vi "aquire single subvi.vi"(8 "Channel":enum16{"Invalid", "Channel 1", "Channel 2"}(ring), 9 "Array":string[](array[string])=["0", "50mv", "100mv", "200mv", "500mv", "1v", "2v", "5v", "10v", "20v", "50v", "0", "0", "0", "0", "0", "0", "0", "0", "0"], 10 "Array 3":string[](array[string])=["5ns", "10ns", "20ns", "50ns", "100ns", "200ns", "500ns", "1us", "2us", "5us", "10us", "20us", "50us", "100us", "200us", "500us", "1ms", "2ms", "5ms", "10ms", "20ms", "50ms", "100ms", "200ms", "500ms", "1s", "2s", "5s", "10s", "20s", "50s", "100s"], 11 "unsigned byte array":u8[](array[numeric])) -> (0 "wave_data(mv)":i32[](array[numeric]), 1 "M":string, 2 "precision":string, 3 "wave_data":i8[](array[numeric]))   [LabVIEW 2023, in "owon.lvlib"]
uses:
  owon.lvlib
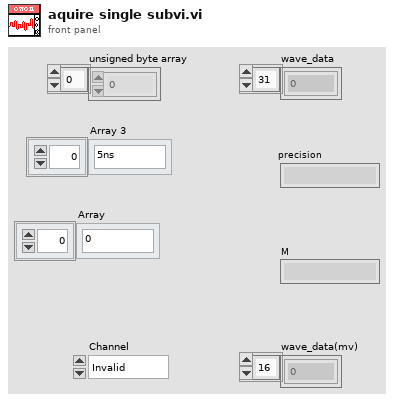
[diagram p1: front panel]
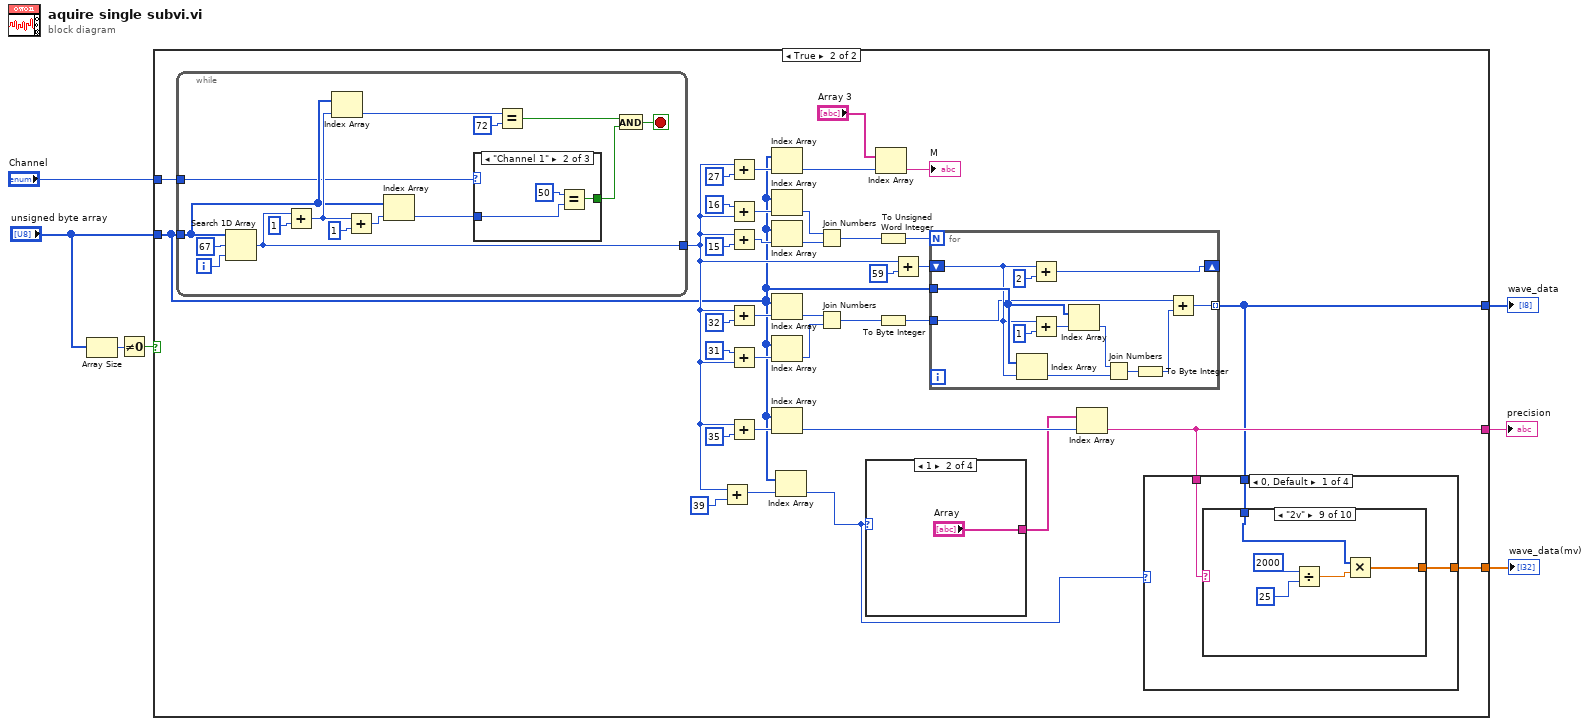
[diagram p0: block diagram]
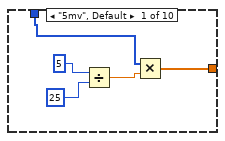
[diagram p3: hidden frame]
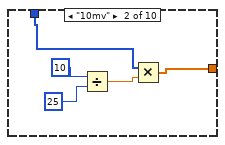
[diagram p4: hidden frame]
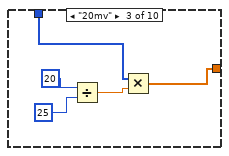
[diagram p5: hidden frame]
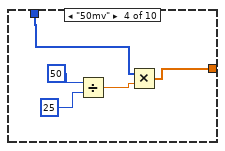
[diagram p6: hidden frame]
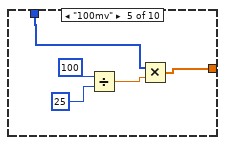
[diagram p7: hidden frame]
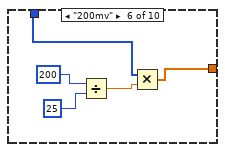
[diagram p8: hidden frame]
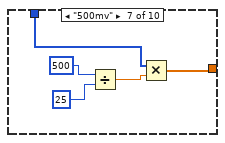
[diagram p9: hidden frame]
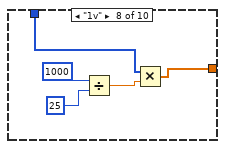
[diagram p10: hidden frame]
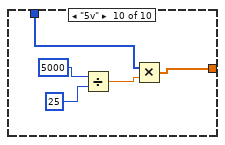
[diagram p11: hidden frame]
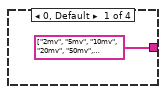
[diagram p15: hidden frame]
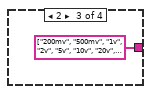
[diagram p16: hidden frame]
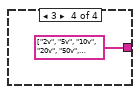
[diagram p17: hidden frame]
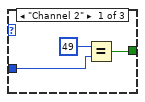
[diagram p18: hidden frame]
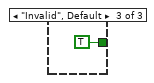
[diagram p19: hidden frame]
diagram:
  n1 = Array Size(array="unsigned byte array") -> (size(s)=w2:i32)
  n2 = Not Equal To 0?(x=w2) -> (x != 0?=w1:bool)
  n3 = case shown="True" w1 {
    tunnel: "unsigned byte array" -> [_ w14]
    tunnel: [_ w11] -> w7
    tunnel: [_ w10] -> w6
    tunnel: [_ w9] -> w5
    tunnel: "Channel" -> [_ w8]
    frame False {
    }
    frame True {
      n4 = while {
        tunnel: w14 -> [w106]
        tunnel: [w110] -> w15
        tunnel: w8 -> [w101]
        i -> [w111]
        stop <- w102 stop-if-true
        n5 = Search 1D Array(1D array=w106, element=u8 67 ("元素"), start index (0)=w111) -> (index of element=w110:i32)
        n6 = Add(x=w110, y=1) -> (x+y=w109:i32)
        n7 = Index Array(array=w106, index=w109) -> (element=w113:u8)
        n8 = Add(x=w109, y=1) -> (x+y=w107:i32)
        n9 = Index Array(array=w106, index=w107) -> (element=w105:u8)
        n10 = case shown="\"Channel 1\"" w101 {
          tunnel: w105 -> [w116 w120 _]
          tunnel: [w117 w119 TRUE] -> w104
          frame "Channel 2" {
            n11 = Equal?(x=u8 49, y=w116) -> (x = y?=w117:bool)
          }
          frame "Channel 1" {
            n12 = Equal?(x=u8 50, y=w120) -> (x = y?=w119:bool)
          }
          frame "Invalid", Default {
          }
        }
        n13 = Equal?(x=w113, y=u8 72 ("元素")) -> (x = y?=w103:bool)
        n14 = And(x=w103, y=w104) -> (x .and. y?=w102:bool)
      }
      n15 = Add(x=w15, y=39) -> (x+y=w17:i32)
      n16 = Add(x=w15, y=27) -> (x+y=w19:i32)
      n17 = Add(x=16 ("索引"), y=w15) -> (x+y=w37:i32)
      n18 = Add(x=w15, y=15 ("索引")) -> (x+y=w39:i32)
      n19 = Add(x=w15, y=32) -> (x+y=w28:i32)
      n20 = Add(x=31, y=w15) -> (x+y=w30:i32)
      n21 = Add(x=w15, y=35) -> (x+y=w22:i32)
      n22 = Index Array(array=w14, index=w19) -> (element=w18:u8)
      n23 = Index Array(array=w14, index=w37) -> (element=w40:u8)
      n24 = Index Array(array=w14, index=w39) -> (element=w41:u8)
      n25 = Index Array(array=w14, index=w28) -> (element=w25:u8)
      n26 = Index Array(array=w14, index=w30) -> (element=w26:u8)
      n27 = Index Array(array=w14, index=w22) -> (element=w21:u8)
      n28 = Index Array(array=w14, index=w17) -> (element=w12:u8)
      n29 = Join Numbers(hi=w40, lo=w41) -> ((hi.lo)=w42:u16)
      n30 = Join Numbers(hi=w25, lo=w26) -> ((hi.lo)=w24:u16)
      n31 = case shown="1" w12 {
        tunnel: [string[] ["2mv", "5mv", "10mv", "20mv", "50mv", "100mv", "200mv", "500mv", "1v", "2v", "5v", "10v", "0", "0", "0", "0", "0", "0", "0", "0"] ("Array 2") "Array" string[] ["200mv", "500mv", "1v", "2v", "5v", "10v", "20v", "50v", "100v", "200v", "500v", "1kv", "0", "0", "0", "0", "0", "0", "0", "0"] ("Array 4") string[] ["2v", "5v", "10v", "20v", "50v", "100v", "200v", "500v", "1kv", "2kv", "5kv", "10kv", "0", "0", "0", "0", "0", "0", "0", "0"] ("Array 5")] -> w13
        frame 0, Default {
        }
        frame 1 {
        }
        frame 2 {
        }
        frame 3 {
        }
      }
      n32 = Index Array(array="Array 3", index=w18) -> (element=→"M":string)
      n33 = To Unsigned Word Integer(number=w42) -> (unsigned 16bit integer=w43:u16)
      n34 = To Byte Integer(number=w24) -> (8bit integer=w33:i8)
      n35 = Add(x=w15, y=59) -> (x+y=w32:i32)
      n36 = for {
        N: w43 -> [_]
        tunnel: w14 -> [w134]
        shift-right: [w131] -> _
        shift-left: w32 -> [w130]
        tunnel: [w126] -> w10 mode=indexing
        tunnel: w33 -> [w123]
        n37 = Index Array(array=w134, index=w130) -> (element=w124:u8)
        n38 = Add(x=w130, y=2) -> (x+y=w131:i32)
        n39 = Add(x=w130, y=1) -> (x+y=w133:i32)
        n40 = Index Array(array=w134, index=w133) -> (element=w125:u8)
        n41 = Join Numbers(hi=w125, lo=w124) -> ((hi.lo)=w128:u16)
        n42 = To Byte Integer(number=w128) -> (8bit integer=w127:i8)
        n43 = Add(x=w123, y=w127) -> (x+y=w126:i8)
      }
      n44 = Index Array(array=w13, index=w21) -> (element=w11:string)
      n45 = case shown="0, Default" w12 {
        tunnel: w11 -> [w46 _ _ _]
        tunnel: w10 -> [w45 _ _ _]
        tunnel: [w44 _ _ _] -> w9
        frame 0, Default {
          n46 = case shown="\"2v\"" w46 {
            tunnel: w45 -> [w48 w53 w58 w63 w68 w73 w78 w83 w88 w93]
            tunnel: [w47 w52 w57 w62 w67 w72 w77 w82 w87 w92] -> w44
            frame "5mv", Default {
              n47 = Divide(x=5, y=25) -> (x/y=w49:dbl)
              n48 = Multiply(x=w48, y=w49) -> (x*y=w47:dbl[])
            }
            frame "10mv" {
              n49 = Divide(x=10, y=25) -> (x/y=w56:dbl)
              n50 = Multiply(x=w53, y=w56) -> (x*y=w52:dbl[])
            }
            frame "20mv" {
              n51 = Divide(x=20, y=25) -> (x/y=w61:dbl)
              n52 = Multiply(x=w58, y=w61) -> (x*y=w57:dbl[])
            }
            frame "50mv" {
              n53 = Divide(x=50, y=25) -> (x/y=w66:dbl)
              n54 = Multiply(x=w63, y=w66) -> (x*y=w62:dbl[])
            }
            frame "100mv" {
              n55 = Divide(x=100, y=25) -> (x/y=w71:dbl)
              n56 = Multiply(x=w68, y=w71) -> (x*y=w67:dbl[])
            }
            frame "200mv" {
              n57 = Divide(x=200, y=25) -> (x/y=w76:dbl)
              n58 = Multiply(x=w73, y=w76) -> (x*y=w72:dbl[])
            }
            frame "500mv" {
              n59 = Divide(x=500, y=25) -> (x/y=w81:dbl)
              n60 = Multiply(x=w78, y=w81) -> (x*y=w77:dbl[])
            }
            frame "1v" {
              n61 = Divide(x=1000, y=25) -> (x/y=w86:dbl)
              n62 = Multiply(x=w83, y=w86) -> (x*y=w82:dbl[])
            }
            frame "2v" {
              n63 = Divide(x=2000, y=25) -> (x/y=w91:dbl)
              n64 = Multiply(x=w88, y=w91) -> (x*y=w87:dbl[])
            }
            frame "5v" {
              n65 = Divide(x=5000, y=25) -> (x/y=w96:dbl)
              n66 = Multiply(x=w93, y=w96) -> (x*y=w92:dbl[])
            }
          }
        }
        frame 1 {
        }
        frame 2 {
        }
        frame 3 {
        }
      }
    }
  }
  "precision" <- w7
  "wave_data" <- w6
  "wave_data(mv)" <- w5
